vi "Update View Dict.vi"(0 "Controller in":refnum<class "Controller.lvclass">, 1 "View Name":string, 2 "Exclude From Broadcast (F)":bool, 3 "Receive Only (F)":bool, 4 "Paused (F)":bool, 5 "error in (no error)":errorcluster) -> (14 "Controller out":refnum<class "Controller.lvclass">, 16 "View Enququer":refnum<class "Message Enqueuer.lvclass">, 19 "error out":errorcluster)   [LabVIEW 2023, in "MVC Actors.lvlib" / "Controller.lvclass"]
uses:
  Controller.lvclass
  <vilib>/ActorFramework/Message Enqueuer/Message Enqueuer.lvclass
  Controller.lvclass/Controller.ctl
  View Details.ctl
  View Messages/Write Receive Only Msg/Write Receive Only Msg.lvclass
  View Messages/Write Paused Msg/Write Paused Msg.lvclass
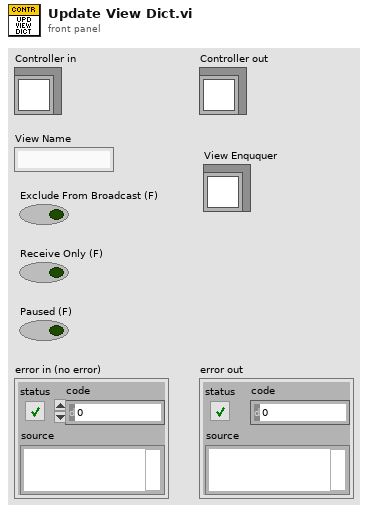
[diagram p1: front panel]
types:
  T1 = typedef "MVC Actors.lvlib/Controller.lvclass/View Details.ctl" = cluster{"Exclude From Broadcast":bool, "Receive Only":bool, "Paused":bool, "View Enqueuer":refnum<class "Message Enqueuer.lvclass">}
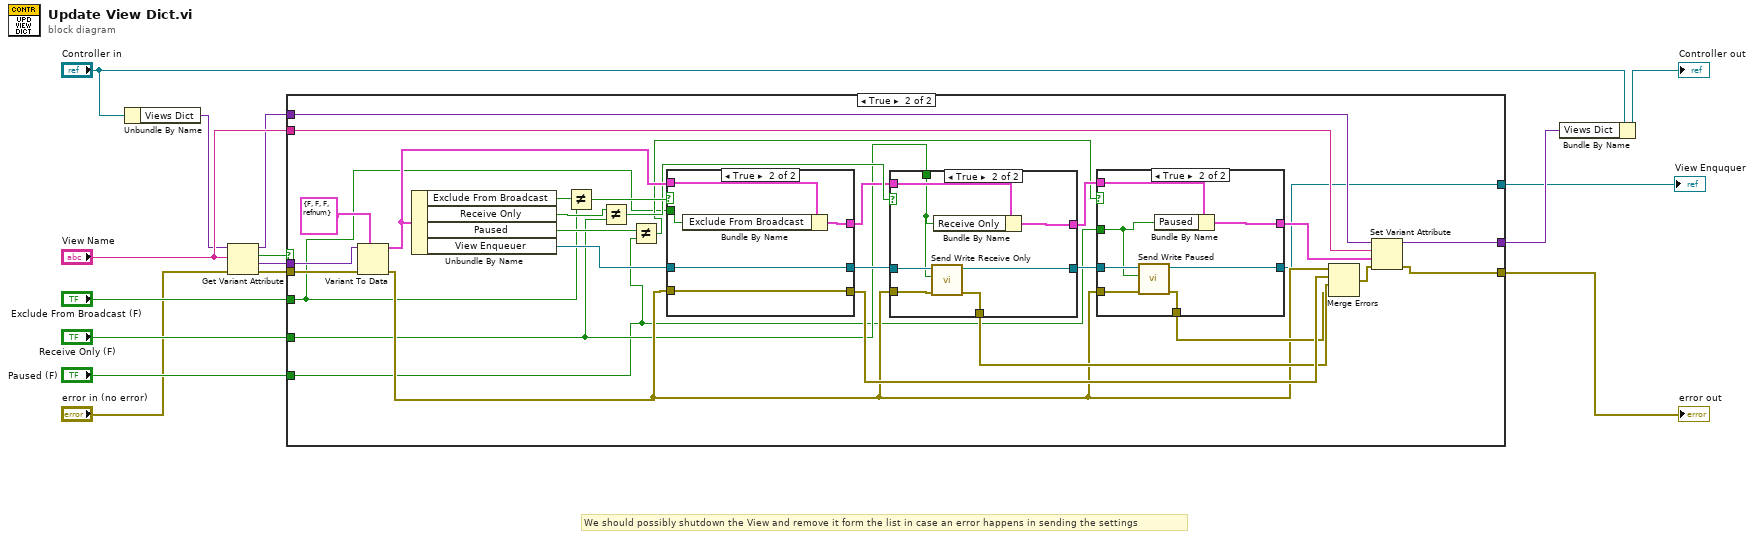
[diagram p0: block diagram]
diagram:
  # "We should possibly shutdown the View and remove it form the list in case an error happens in sending the settings"
  n1 = Unbundle By Name("Controller in") -> ("Views Dict"=w2:variant)
  n2 = Get Variant Attribute(Variant=w2, name="View Name", error in="error in (no error)") -> (duplicate Variant=w13:variant, found=w3:bool, value=w4:variant, error out=w5:errorcluster)  [unwired: 1 in]
  n3 = case shown="True" w3 {
    tunnel: w4 -> [_ w45]
    tunnel: w5 -> [w17 w46]
    tunnel: [w17 w26] -> w7
    tunnel: "Exclude From Broadcast (F)" -> [_ w20]
    tunnel: "Receive Only (F)" -> [_ w19]
    tunnel: "Paused (F)" -> [_ w18]
    tunnel: w13 -> [w16 w32]
    tunnel: "View Name" -> [_ w31]
    tunnel: [w16 w25] -> w15
    tunnel: [_ w21] -> w1
    frame False {
    }
    frame True {
      n4 = Variant To Data(error in=w46, type=T1 {"Exclude From Broadcast"=FALSE, "Receive Only"=FALSE, "Paused"=FALSE, "View Enqueuer"=refnum} ("Message Enqueuer"), Variant=w45) -> (data=w42:T1, error out=w23:errorcluster)
      n5 = Unbundle By Name(w42) -> ("Exclude From Broadcast"=w24:bool, "Receive Only"=w37:bool, "Paused"=w33:bool, "View Enqueuer"=w43:refnum<class "Message Enqueuer.lvclass">)
      n6 = Not Equal?(x=w24, y=w20) -> (x != y?=w41:bool)
      n7 = Not Equal?(x=w37, y=w19) -> (x != y?=w40:bool)
      n8 = Not Equal?(x=w33, y=w18) -> (x != y?=w34:bool)
      n9 = case shown="True" w41 {
        tunnel: w43 -> [w68 w74]
        tunnel: [w68 w74] -> w39
        tunnel: w42 -> [w69 w73]
        tunnel: [w69 w72] -> w38
        tunnel: w20 -> [_ w71]
        tunnel: w23 -> [w67 w70]
        tunnel: [w67 w70] -> w29
        frame False {
        }
        frame True {
          n10 = Bundle By Name(cluster=w73, "Exclude From Broadcast"=w71) -> (w72:T1)
        }
      }
      n11 = case shown="True" w40 {
        tunnel: w39 -> [w58 w66]
        tunnel: [w58 w65] -> w36
        tunnel: w38 -> [w59 w64]
        tunnel: [w59 w63] -> w35
        tunnel: w19 -> [_ w60]
        tunnel: w23 -> [w57 w62]
        tunnel: [w57 w61] -> w28
        frame False {
        }
        frame True {
          n12 = call "Send Write Receive Only.vi"("error in (no error)"=w62, "Receive Only"=w60, "Message Enqueuer in"=w66) -> ("error out"=w61:errorcluster, "Message Enqueuer out"=w65:refnum<class "Message Enqueuer.lvclass">)  [unwired: 7 in]
          n13 = Bundle By Name(cluster=w64, "Receive Only"=w60) -> (w63:T1)
        }
      }
      n14 = case shown="True" w34 {
        tunnel: w36 -> [w48 w56]
        tunnel: [w48 w55] -> w21
        tunnel: w35 -> [w49 w54]
        tunnel: [w49 w53] -> w30
        tunnel: w23 -> [w47 w52]
        tunnel: w18 -> [_ w50]
        tunnel: [w47 w51] -> w27
        frame False {
        }
        frame True {
          n15 = call "Send Write Paused.vi"("error in (no error)"=w52, "Paused"=w50, "Message Enqueuer in"=w56) -> ("error out"=w51:errorcluster, "Message Enqueuer out"=w55:refnum<class "Message Enqueuer.lvclass">)  [unwired: 7 in]
          n16 = Bundle By Name(cluster=w54, "Paused"=w50) -> (w53:T1)
        }
      }
      n17 = Merge Errors(w23, w29, w28, w27) -> (w22:errorcluster)
      n18 = Set Variant Attribute(Variant=w32, name=w31, value=w30, error in=w22) -> (Variant out=w25:variant, error out=w26:errorcluster)  [unwired: 1 out]
    }
  }
  "error out" <- w7
  "View Enququer" <- w1
  n19 = Bundle By Name(cluster="Controller in", "Views Dict"=w15) -> (→"Controller out":refnum<class "Controller.lvclass">)
